vi "Initialize UI core.vi"(8 "error in (no error)":errorcluster, 11 "Window in":refnum<class "Window.lvclass">) -> (0 "error out":errorcluster, 1 "Autoshow?":bool, 2 "Panel Updater":refnum<class "Panel Updater.lvclass">, 3 "Window out":refnum<class "Window.lvclass">)   [LabVIEW 2017, in "MGI-Panel Manager.lvlib" / "Window.lvclass"]
doc: "Opens the FP as hidden and centers it.\n\n----\nPlease see the following web address for additional documentation and tutorial information:\nhttp://www.mooregoodideas.com/mgi-panel-manager/\n\nAuthor: Derek Trepanier\n\nCopyright (c) 2018, Moore Good Ideas, Inc.\n\nAll rights reserved.\n\nRedistribution and use in source and binary forms, with or without modification, are permitted provided that the following conditions are met:\n\n * Redistributions of source code must retain the above copyright notice, this list of conditions and the following disclaimer.\n * Redistributions in binary form must reproduce the above copyright notice, this list of conditions and the following disclaimer in the documentation and/or other materials provided with the distribution.\n * Neither the name of Moore Good Ideas, Inc. nor the names of its contributors may be used to endorse or promote products derived from this software without specific prior written permission.\n\nTHIS SOFTWARE IS PROVIDED BY THE COPYRIGHT HOLDERS AND CONTRIBUTORS \"AS IS\" AND ANY EXPRESS OR IMPLIED WARRANTIES, INCLUDING, BUT NOT LIMITED TO, THE IMPLIED WARRANTIES OF MERCHANTABILITY AND FITNESS FOR A PARTICULAR PURPOSE ARE DISCLAIMED. IN NO EVENT SHALL THE COPYRIGHT OWNER OR CONTRIBUTORS BE LIABLE FOR ANY DIRECT, INDIRECT, INCIDENTAL, SPECIAL, EXEMPLARY, OR CONSEQUENTIAL DAMAGES (INCLUDING, BUT NOT LIMITED TO, PROCUREMENT OF SUBSTITUTE GOODS OR SERVICES; LOSS OF USE, DATA, OR PROFITS; OR BUSINESS INTERRUPTION) HOWEVER CAUSED AND ON ANY THEORY OF LIABILITY, WHETHER IN CONTRACT, STRICT LIABILITY, OR TORT (INCLUDING NEGLIGENCE OR OTHERWISE) ARISING IN ANY WAY OUT OF THE USE OF THIS SOFTWARE, EVEN IF ADVISED OF THE POSSIBILITY OF SUCH DAMAGE."
uses:
  Window.lvclass
  D:/software/LabView_PanelManager/panel-manager/Source/Panel/Panel.lvclass
  Panel Updater/Panel Updater.lvclass
  Panel.lvclass/Panel.ctl
  Window.lvclass/Window.ctl
  Panel Updater/Window Updater/Window Updater.lvclass/Window Updater.ctl
  Panel Updater/Window Updater/Window Updater.lvclass
  D:/software/LabView_PanelManager/panel-manager/Source/Panel Updater/Panel Updater.lvclass
  Panel.lvclass
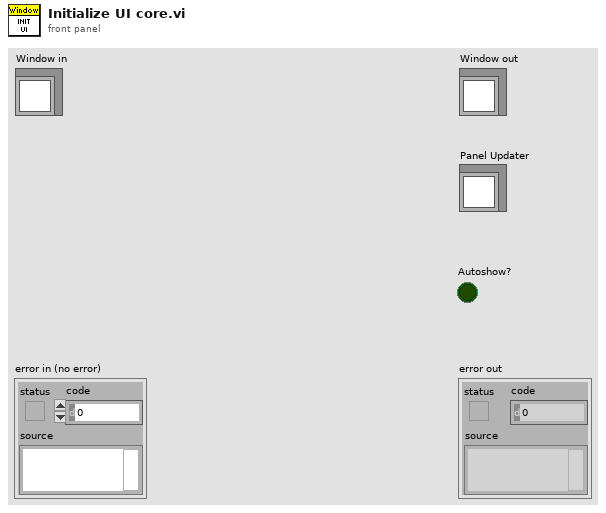
[diagram p1: front panel]
types:
  T1 = enum32{"Invalid", "Standard", "Closed", "Hidden", "Minimized", "Maximized"}
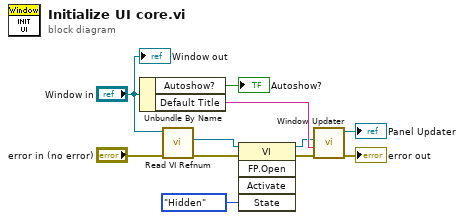
[diagram p0: block diagram]
diagram:
  n1 = Unbundle By Name("Window in") -> ("Autoshow?"=→"Autoshow?":bool, "Default Title"=w5:string)
  n2 = call "Read VI Refnum.vi"("error in (no error)"="error in (no error)", "Panel in"="Window in") -> ("error out"=w8:errorcluster, "VI Refnum"=w9:refnum<vi>)  [unwired: 8 in]
  n3 = invoke class="VI" method="FP.Open"(reference=w9, error in=w8, "State"=T1."Hidden") -> (reference out=w4:refnum<vi>, error out=w2:errorcluster)  [unwired: 2 in, 3 out]
  n4 = call "Window Updater.vi"("error in (no error)"=w2, "Default Title"=w5, "Panel"=w4) -> ("error out"=→"error out":errorcluster, "Window Updater out"=→"Panel Updater":refnum<class "Window Updater.lvclass">)  [unwired: 7 in]
  "Window out" <- "Window in"
